vi "Get alarms from PGserver.vi"(6 "conninfo":T1={"host"="localhost", "port"="5432", "client_encoding"="WIN1251", "dbname"="data", "user"="postgres", "password"=""}, 8 "error in":errorcluster, 9 "LevelTable":string[](array[string]), 10 "ALRParamTable":string="f_alr_3", 11 "fcodealr_full":string[](array[string])) -> (0 "error out":errorcluster, 1 "ALRParameters table":u32[][](array[numeric])=[[0, 0, 0, 0, 0, 0, 0], [1, 11, 5000, 5000, 0, 0, 3], [2, 11, 5000, 5000, 0, 2, 3], [3, 11, 5000, 5000, 0, 3, 3], [4, 11, 1000, 0, 0, 4, 0], [5, 1, 5000, 5000, 0, 1, 3], [6, 1, 5000, 5000, 0, 0, 3], [7, 1, 5000, 5000, 0, 2, 3], [8, 1, 5000, 30000, 0, 3, 3], [9, 1, 1000, 0, 0, 4, 0], [10, 2, 5000, 5000, 0, 1, 3], [11, 2, 5000, 5000, 0, 0, 3], [12, 2, 5000, 5000, 0, 2, 3], [13, 2, 5000, 30000, 0, 3, 3], [14, 2, 1000, 0, 0, 4, 0], [15, 10, 5000, 5000, 0, 0, 3], [16, 10, 5000, 5000, 0, 2, 3], [17, 10, 5000, 5000, 0, 3, 3], [18, 10, 1000, 0, 0, 4, 0], [19, 3, 5000, 5000, 0, 2, 3], [20, 3, 5000, 5000, 0, 3, 3], [21, 3, 1000, 0, 0, 4, 0], [22, 4, 5000, 5000, 0, 2, 3], [23, 4, 5000, 5000, 0, 3, 3], [24, 4, 1000, 0, 0, 4, 0], [25, 5, 5000, 5000, 0, 2, 3], [26, 5, 5000, 5000, 0, 3, 3], [27, 5, 1000, 0, 0, 4, 0], [28, 6, 5000, 5000, 0, 2, 3], [29, 6, 1000, 0, 0, 4, 0], [30, 7, 1000, 0, 0, 4, 0], [31, 8, 1000, 0, 0, 4, 0], [32, 9, 5000, 5000, 0, 0, 3]], 2 "ALR type":T3[](array[typedef]), 3 "ALR code":T4[](array[typedef]), 4 "ALRNames":string[][](array[string])=[["", "Перелив в емкости охлажденной воды", "Уровень в емкости охлажденной воды низкий", "Уровень в емкости охлажденной воды аварийно низкий", "Датчик уровня в емкости охлажденной воды неисправен", "Давление после насосов градирни аварийно высокое", "Давление после насосов градирни высокое", "Давление после насосов градирни низкое", "Давление после насосов градирни аварийно низкое", "Датчик давления после насосов градирни неисправен", "Давление перед градирней аварийно высокое", "Давление перед градирней высокое", "Давление перед градирней низкое", "Давление перед градирней аварийно низкое", "Датчик давления перед градирней неисправен", "Перелив в емкости дистиллята", "Уровень в емкости дистиллята низкий", "Уровень в емкости дистиллята аварийно низкий", "Датчик уровеня в емкости дистиллята неисправен", "Давление после насосов дистиллята низкое", "Давление после насосов дистиллята аварийно низкое", "Датчик давления после насосов дистиллята неисправен", "Давление дистиллята перед реактором низкое", "Давление дистиллята перед реактором аварийно низкое", "Датчик давления перед реактором неисправен", "Давление после насоса агломератора низкое", "Давление после насоса агломератора аварийно низкое", "Датчик давления после насоса агломератора неисправен", "Температура после градирни низкая", "Датчик температуры после градирни неисправен", "Датчик температуры перед градирней неисправен", "Датчик температуры дистиллята после насосов неисправен", "Температура дистиллята перед реактором высокая"]], 5 "ALRLevel table":i32[][](array[numeric])=[[0, 0, 0, 0, 0, 0, 0], [1, 11, 5000, 5000, 0, 0, 3], [2, 11, 5000, 5000, 0, 2, 3], [3, 11, 5000, 5000, 0, 3, 3], [4, 11, 1000, 0, 0, 4, 0], [5, 1, 5000, 5000, 0, 1, 3], [6, 1, 5000, 5000, 0, 0, 3], [7, 1, 5000, 5000, 0, 2, 3], [8, 1, 5000, 30000, 0, 3, 3], [9, 1, 1000, 0, 0, 4, 0], [10, 2, 5000, 5000, 0, 1, 3], [11, 2, 5000, 5000, 0, 0, 3], [12, 2, 5000, 5000, 0, 2, 3], [13, 2, 5000, 30000, 0, 3, 3], [14, 2, 1000, 0, 0, 4, 0], [15, 10, 5000, 5000, 0, 0, 3], [16, 10, 5000, 5000, 0, 2, 3], [17, 10, 5000, 5000, 0, 3, 3], [18, 10, 1000, 0, 0, 4, 0], [19, 3, 5000, 5000, 0, 2, 3], [20, 3, 5000, 5000, 0, 3, 3], [21, 3, 1000, 0, 0, 4, 0], [22, 4, 5000, 5000, 0, 2, 3], [23, 4, 5000, 5000, 0, 3, 3], [24, 4, 1000, 0, 0, 4, 0], [25, 5, 5000, 5000, 0, 2, 3], [26, 5, 5000, 5000, 0, 3, 3], [27, 5, 1000, 0, 0, 4, 0], [28, 6, 5000, 5000, 0, 2, 3], [29, 6, 1000, 0, 0, 4, 0], [30, 7, 1000, 0, 0, 4, 0], [31, 8, 1000, 0, 0, 4, 0], [32, 9, 5000, 5000, 0, 0, 3]])   [LabVIEW 2019, in "Alarms.lvlib"]
uses:
  Alarms.lvlib
  Ctl/ALR code.ctl
  Ctl/ALR type.ctl
  Database/ctl/Coninfo.ctl
  Ctl/ALRColumns.ctl
  Database/PostgreSQL2LabVIEW/libpqlv/src/PQfinish.vi
  Database/PostgreSQL2LabVIEW/libpqlv/src/PQconnectdb.vi
  Database/PostgreSQL2LabVIEW/libpqlv/src/PQerrorMessage.vi
  Database/PostgreSQL2LabVIEW/libpqlv/src/PQstatus.vi
  <vilib>/dlg_ctls.llb/Space Constant.vi
  Database/Progress.vi
  Database/PostgreSQL.lvlib
  Database/PostgreSQL2LabVIEW/libpqUtility/libpqutility.lvlib
  Database/PostgreSQL2LabVIEW/libpqUtility64/libpqutility64.lvlib
panel:
  out "PQStatus":T2(ring)
  # "fnum"
  # "alr_ton"
  # "alr_toff"
  # "n_repeat"
  # "fcodealr_full"
  # "alr_name"
  # "fcode_full"
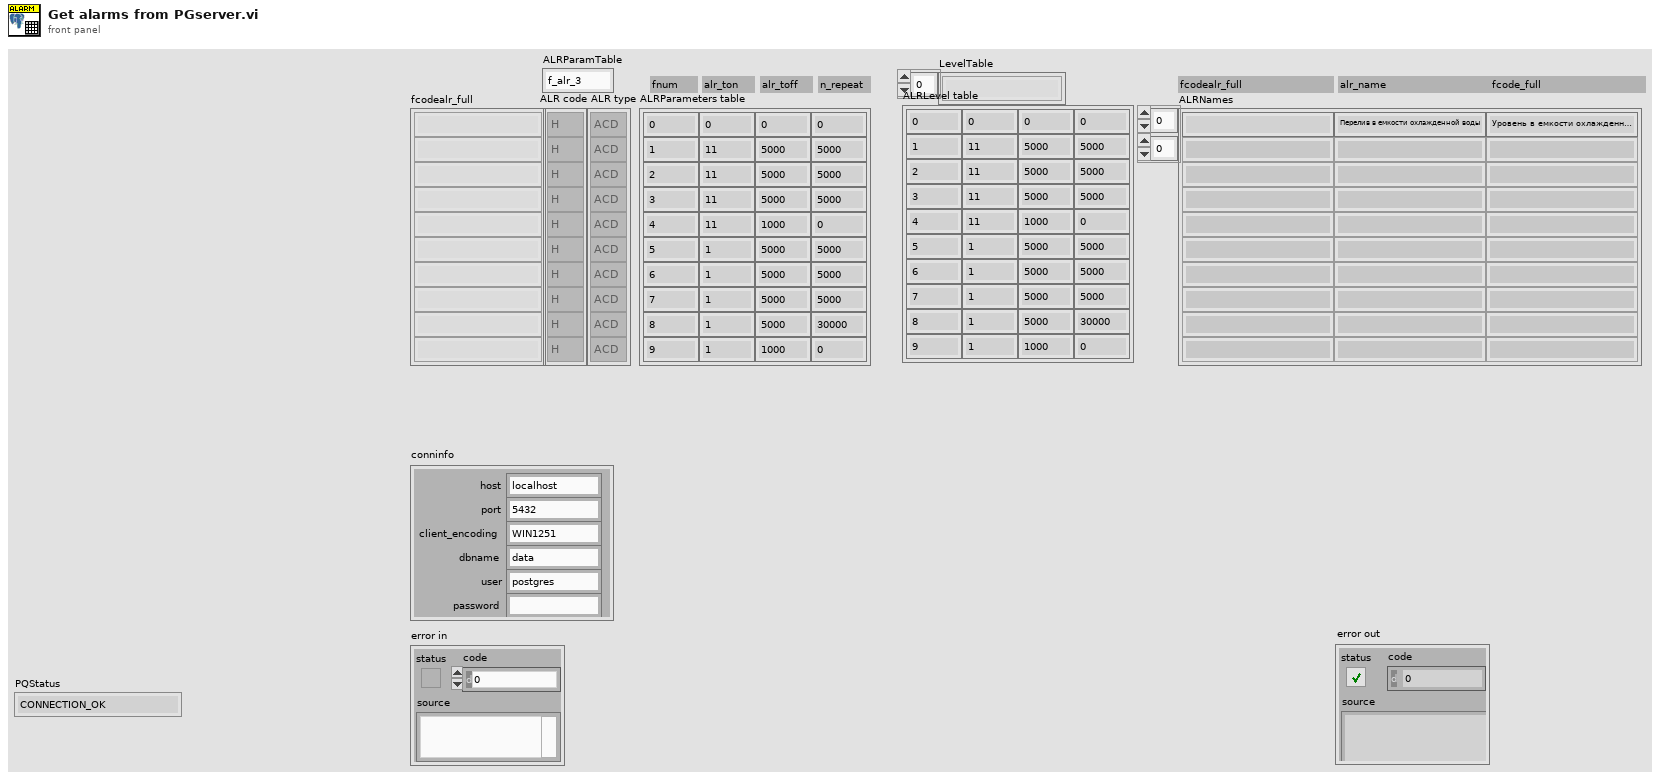
[diagram p1: front panel]
types:
  T1 = typedef "PostgreSQL.lvlib/Coninfo.ctl" = cluster{"host":string, "port":string, "client_encoding":string, "dbname":string, "user":string, "password":string}
  T2 = enum32{"CONNECTION_OK", "CONNECTION_BAD", "CONNECTION_STARTED", "CONNECTION_MADE", "CONNECTION_AWAITING_RESPONSE", "CONNECTION_AUTH_OK", "CONNECTION_SETENV", "CONNECTION_SSL_STARTUP", "CONNECTION_NEEDED"}
  T3 = typedef "Alarms.lvlib/ALR type.ctl" = enum16{"ACD", "ACDR", "ALRN", "ALR"}
  T4 = typedef "Alarms.lvlib/ALR code.ctl" = enum16{"CONN", "H", "HH", "L", "LL", "SERR", "ON", "OFF", "XM19", "XM24", "XM47", "XM51", "XM52", "XM53", "XM54", "XM55", "XM56", "XM61", "XM62", "XM63", "XM64", "XM65", "XM66"}
  T5 = typedef "Alarms.lvlib/ALRColumns.ctl" = enum16{"alr_ton", "alr_toff", "n_repeat", "fcodealr", "alr_type", "alrname", "fcode_full"}
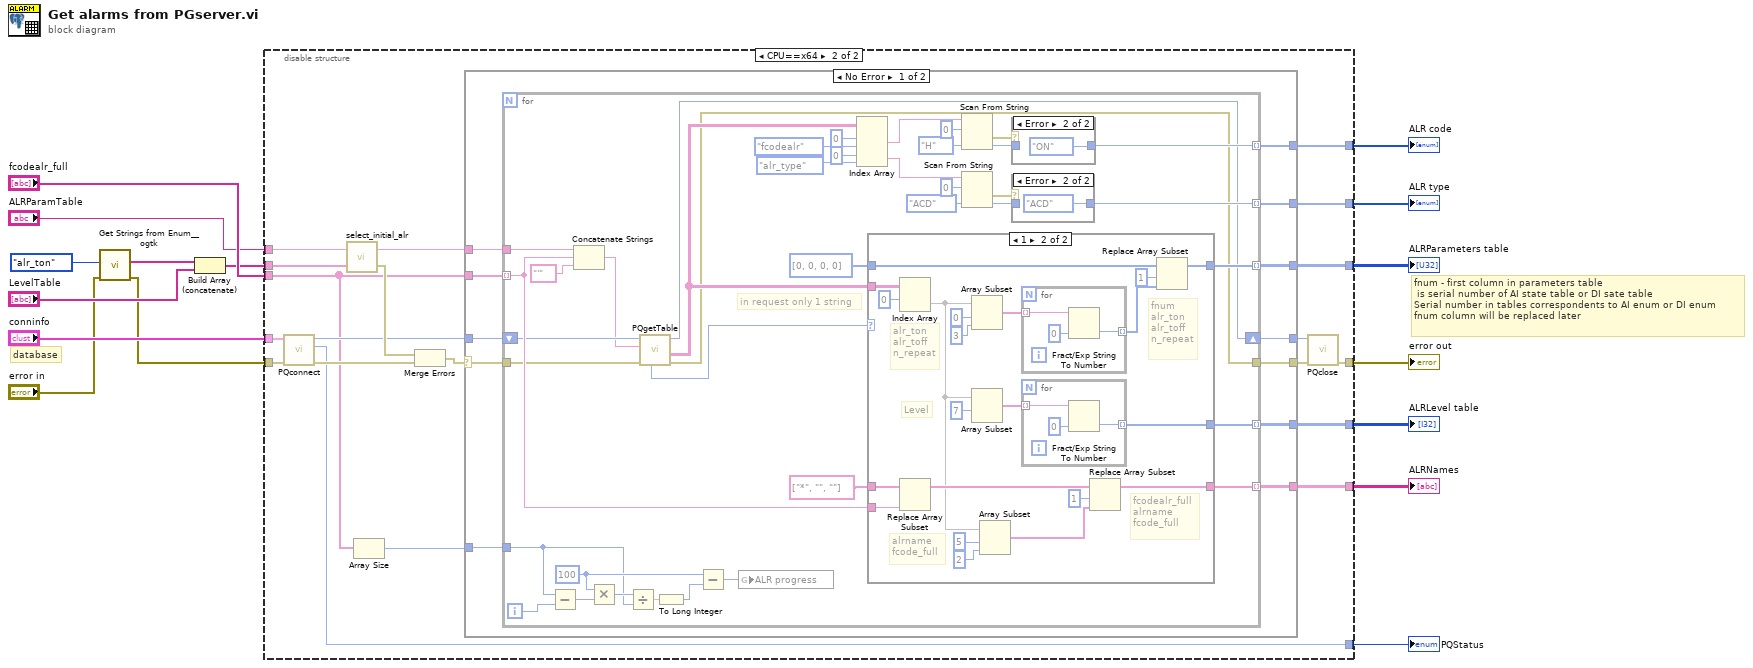
[diagram p0: block diagram]
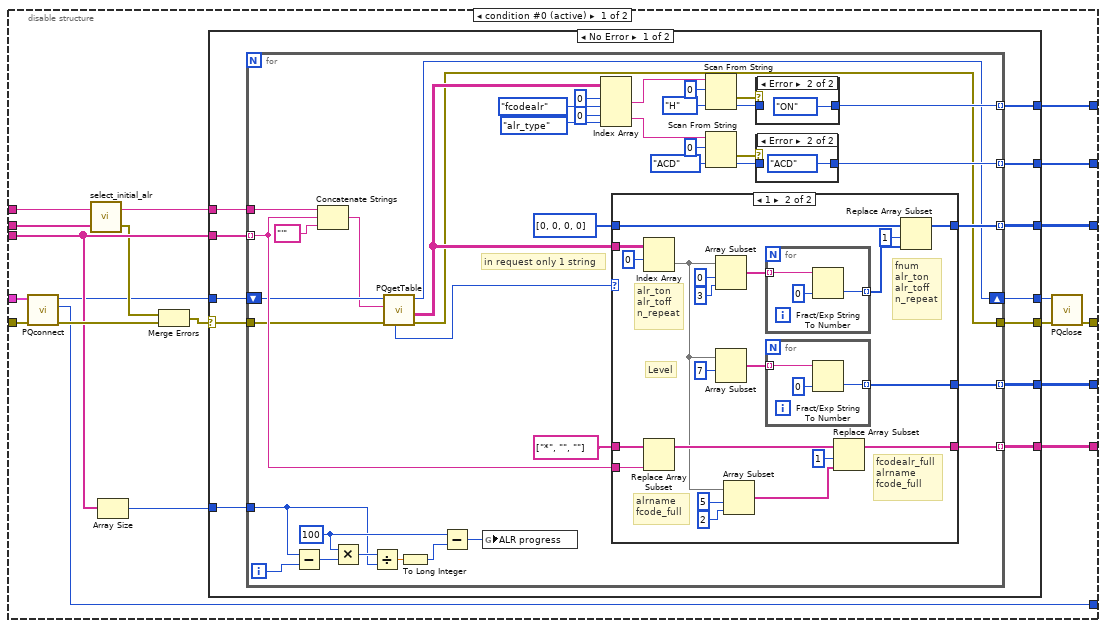
[diagram p2: hidden frame]
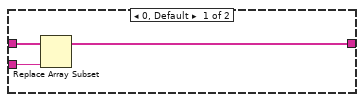
[diagram p3: hidden frame]
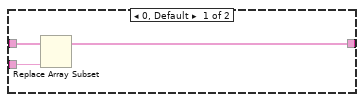
[diagram p7: hidden frame]
diagram:
  # "fnum - first column in parameters table\n is serial number of AI state table or DI sate table\nSerial number in tables correspondents to AI enum or DI enum\nfnum column will be replaced later"
  # "database"
  n1 = call <userlib>:"Get Strings from Enum__ogtk.vi"("error in (no error)"="error in", "Enum"=ALRColumns."alr_ton" ("ALRColumns")) -> ("error out"=w2:errorcluster, "Enum Strings"=w1:string[])  [unwired: 6 in, 2 out]
  n2 = Build Array (concatenate)(w1, "LevelTable") -> (w7:string[])
  n3 = disable-structure shown="CPU==x64" {
    disable-tunnel: "fcodealr_full" -> [w35 w133]
    disable-tunnel: [w34 w126] -> w15
    disable-tunnel: "ALRParamTable" -> [w33 w135]
    disable-tunnel: [w32 w125] -> w13
    disable-tunnel: [w31 w124] -> w12
    disable-tunnel: [w30 w127] -> w11
    disable-tunnel: [w29 w129] -> w10
    disable-tunnel: "conninfo" -> [w28 w132]
    disable-tunnel: w2 -> [w26 w131]
    disable-tunnel: w7 -> [w25 w134]
    disable-tunnel: [w24 w128] -> w6
    disable-tunnel: [w23 w130] -> w5
    frame condition #0 (active) {
      n4 = call "PQconnect.vi"("error in (no error)"=w26, "conninfo"=w28) -> ("error out"=w36:errorcluster, "PQStatus"=w23:T2, "conn"=w18:u32)  [unwired: 7 in]
      n5 = call "select_initial_alr.vi"("Column table"=w25, "table"=w33) -> ("Data to write"=w20:errorcluster, "parameters"=w21:string)
      n6 = Array Size(array=w35) -> (size(s)=w22:i32)
      n7 = Merge Errors(w20, w36) -> (w19:errorcluster)
      n8 = case shown="No Error" w19 {
        selector: w19 -> [w46 w123]
        tunnel: w35 -> [w44 _]
        tunnel: [w48 _] -> w34
        tunnel: [w47 _] -> w29
        tunnel: w22 -> [w45 _]
        tunnel: w18 -> [w43 w122]
        tunnel: w21 -> [w42 _]
        tunnel: [w41 _] -> w31
        tunnel: [w40 _] -> w32
        tunnel: [w39 w123] -> w27
        tunnel: [w38 _] -> w24
        tunnel: [w37 w122] -> w17
        frame No Error {
          n9 = for {
            tunnel: [w65] -> w47 mode=indexing
            tunnel: [w62] -> w48 mode=indexing
            tunnel: w46 -> [w56]
            tunnel: w45 -> [w78]
            tunnel: w44 -> [w61] mode=indexing
            tunnel: w42 -> [w87]
            tunnel: [w64] -> w41 mode=indexing
            tunnel: [w63] -> w40 mode=indexing
            tunnel: [w54] -> w39
            tunnel: [w52] -> w38 mode=indexing
            shift-right: [w51] -> w37
            shift-left: w43 -> [w58]
            i -> [w79]
            w83 = 100 ("y")
            # "in request only 1 string"
            n10 = Subtract(x=w78, y=w79) -> (x-y=w82:i32)
            n11 = Concatenate Strings(w87, w61, "'" ("table")) -> (w57:string)
            n12 = Multiply(x=w83, y=w82) -> (x*y=w85:i32)
            n13 = Divide(x=w85, y=w78) -> (x/y=w81:dbl)
            n14 = call "PQgetTable.vi"("error in"=w56, "query"=w57, "conn"=w58) -> ("error out"=w54:errorcluster, "Data"=w55:string[][], "conn_out"=w51:u32, "PQnTuples"=w53:i32)  [unwired: 4 in, 1 out]
            n15 = To Long Integer(number=w81) -> (32bit integer=w80:i32)
            n16 = Subtract(x=w83, y=w80) -> (x-y=w84:i32)
            n17 = global write "Progress.vi" "ALR progress"(w84) -> ()
            n18 = Index Array(array=w55, index (row) #1=0 ("disabled index (row)"), index (col) #1=ALRColumns."fcodealr" ("ALRColumns"), index (row) #2=0 ("disabled index (row)"), index (col) #2=ALRColumns."alr_type" ("ALRColumns")) -> (element #1=w74:string, element #2=w68:string)
            n19 = case shown="1" w53 {
              tunnel: [_ w98] -> w62
              tunnel: w55 -> [_ w111]
              tunnel: [w88 w102] -> w65
              tunnel: w61 -> [w90 w106]
              tunnel: string[] ["*", "", ""] ("appended array") -> [w89 w107]
              tunnel: u32[] [0, 0, 0, 0] ("appended array") -> [_ w101]
              tunnel: [_ w91] -> w52
              frame 0, Default {
                n20 = Replace Array Subset(array=w89, new element=w90) -> (w88:string[])  [unwired: 1 in]
              }
              frame 1 {
                # "fnum\nalr_ton\nalr_toff\nn_repeat"
                # "fcodealr_full\nalrname\nfcode_full"
                # "alrname\nfcode_full"
                # "Level"
                # "alr_ton\nalr_toff\nn_repeat"
                n21 = Index Array(array=w111, index (row)=0) -> (element=w93:string[])  [unwired: 1 in]
                n22 = Replace Array Subset(array=w107, new element=w106) -> (w105:string[])  [unwired: 1 in]
                n23 = Array Subset(array=w93, index=0, length=3) -> (w95:string[])
                n24 = Array Subset(array=w93, index=7) -> (w92:string[])  [unwired: 1 in]
                n25 = Array Subset(array=w93, index=5, length=2) -> (w104:string[])
                n26 = for {
                  tunnel: w95 -> [w117] mode=indexing
                  tunnel: [w116] -> w99 mode=indexing
                  n27 = Fract/Exp String To Number(string=w117, default (0 dbl)=u32 0 ("String")) -> (number=w116:u32)  [unwired: 2 in, 1 out]
                }
                n28 = for {
                  tunnel: w92 -> [w114] mode=indexing
                  tunnel: [w113] -> w91 mode=indexing
                  n29 = Fract/Exp String To Number(string=w114, default (0 dbl)=0 ("String")) -> (number=w113:i32)  [unwired: 2 in, 1 out]
                }
                n30 = Replace Array Subset(array=w105, new element=w104, index=1) -> (w102:string[])
                n31 = Replace Array Subset(array=w101, new element=w99, index=1) -> (w98:u32[])
              }
            }
            n32 = Scan From String(input string=w74, initial scan location=u32 0, default 1=ALR_code."H" ("ALR code")) -> (error out=w77:errorcluster, output 1=w73:T4)  [unwired: 2 in, 2 out]
            n33 = Scan From String(input string=w68, initial scan location=u32 0, default 1=ALR_type."ACD" ("ALR type")) -> (error out=w70:errorcluster, output 1=w72:T3)  [unwired: 2 in, 2 out]
            n34 = case shown="Error" w77 {
              tunnel: w73 -> [w120 _]
              tunnel: [w120 ALR_code."ON" ("ALR code")] -> w64
              frame No Error {
              }
              frame Error {
              }
            }
            n35 = case shown="Error" w70 {
              tunnel: w72 -> [w118 _]
              tunnel: [w118 ALR_type."ACD" ("ALR type")] -> w63
              frame No Error {
              }
              frame Error {
              }
            }
          }
        }
        frame Error {
        }
      }
      n36 = call "PQclose.vi"("error in (no error)"=w27, "conn"=w17) -> ("error out"=w30:errorcluster)  [unwired: 9 in]
    }
    frame condition #1 {
      n37 = call "PQconnect.vi"("error in (no error)"=w131, "conninfo"=w132) -> ("error out"=w143:errorcluster, "PQStatus"=w130:T2, "conn"=w137:u64)  [unwired: 7 in]
      n38 = call "select_initial_alr.vi"("Column table"=w134, "table"=w135) -> ("Data to write"=w139:errorcluster, "parameters"=w140:string)
      n39 = Array Size(array=w133) -> (size(s)=w141:i32)
      n40 = Merge Errors(w139, w143) -> (w138:errorcluster)
      n41 = case shown="No Error" w138 {
        selector: w138 -> [w153 w230]
        tunnel: w133 -> [w151 _]
        tunnel: [w155 _] -> w126
        tunnel: [w154 _] -> w129
        tunnel: w141 -> [w152 _]
        tunnel: w137 -> [w150 w229]
        tunnel: w140 -> [w149 _]
        tunnel: [w148 _] -> w124
        tunnel: [w147 _] -> w125
        tunnel: [w146 w230] -> w142
        tunnel: [w145 _] -> w128
        tunnel: [w144 w229] -> w136
        frame No Error {
          n42 = for {
            tunnel: [w172] -> w154 mode=indexing
            tunnel: [w169] -> w155 mode=indexing
            tunnel: w153 -> [w163]
            tunnel: w152 -> [w185]
            tunnel: w151 -> [w168] mode=indexing
            tunnel: w149 -> [w194]
            tunnel: [w171] -> w148 mode=indexing
            tunnel: [w170] -> w147 mode=indexing
            tunnel: [w161] -> w146
            tunnel: [w159] -> w145 mode=indexing
            shift-right: [w158] -> w144
            shift-left: w150 -> [w165]
            i -> [w186]
            w190 = 100 ("y")
            # "in request only 1 string"
            n43 = Subtract(x=w185, y=w186) -> (x-y=w189:i32)
            n44 = Concatenate Strings(w194, w168, "'" ("table")) -> (w164:string)
            n45 = Multiply(x=w190, y=w189) -> (x*y=w192:i32)
            n46 = Divide(x=w192, y=w185) -> (x/y=w188:dbl)
            n47 = call "PQgetTable.vi"("error in"=w163, "query"=w164, "conn"=w165) -> ("error out"=w161:errorcluster, "Data"=w162:string[][], "conn_out"=w158:u64, "PQnTuples"=w160:i64)  [unwired: 4 in, 1 out]
            n48 = To Long Integer(number=w188) -> (32bit integer=w187:i32)
            n49 = Subtract(x=w190, y=w187) -> (x-y=w191:i32)
            n50 = global write "Progress.vi" "ALR progress"(w191) -> ()
            n51 = Index Array(array=w162, index (row) #1=0 ("disabled index (row)"), index (col) #1=ALRColumns."fcodealr" ("ALRColumns"), index (row) #2=0 ("disabled index (row)"), index (col) #2=ALRColumns."alr_type" ("ALRColumns")) -> (element #1=w181:string, element #2=w175:string)
            n52 = case shown="1" w160 {
              tunnel: [_ w205] -> w169
              tunnel: w162 -> [_ w218]
              tunnel: [w195 w209] -> w172
              tunnel: w168 -> [w197 w213]
              tunnel: string[] ["*", "", ""] ("appended array") -> [w196 w214]
              tunnel: u32[] [0, 0, 0, 0] ("appended array") -> [_ w208]
              tunnel: [_ w198] -> w159
              frame 0, Default {
                n53 = Replace Array Subset(array=w196, new element=w197) -> (w195:string[])  [unwired: 1 in]
              }
              frame 1 {
                # "fnum\nalr_ton\nalr_toff\nn_repeat"
                # "fcodealr_full\nalrname\nfcode_full"
                # "alrname\nfcode_full"
                # "Level"
                # "alr_ton\nalr_toff\nn_repeat"
                n54 = Index Array(array=w218, index (row)=0) -> (element=w200:string[])  [unwired: 1 in]
                n55 = Replace Array Subset(array=w214, new element=w213) -> (w212:string[])  [unwired: 1 in]
                n56 = Array Subset(array=w200, index=0, length=3) -> (w202:string[])
                n57 = Array Subset(array=w200, index=7) -> (w199:string[])  [unwired: 1 in]
                n58 = Array Subset(array=w200, index=5, length=2) -> (w211:string[])
                n59 = for {
                  tunnel: w202 -> [w224] mode=indexing
                  tunnel: [w223] -> w206 mode=indexing
                  n60 = Fract/Exp String To Number(string=w224, default (0 dbl)=u32 0 ("String")) -> (number=w223:u32)  [unwired: 2 in, 1 out]
                }
                n61 = for {
                  tunnel: w199 -> [w221] mode=indexing
                  tunnel: [w220] -> w198 mode=indexing
                  n62 = Fract/Exp String To Number(string=w221, default (0 dbl)=0 ("String")) -> (number=w220:i32)  [unwired: 2 in, 1 out]
                }
                n63 = Replace Array Subset(array=w212, new element=w211, index=1) -> (w209:string[])
                n64 = Replace Array Subset(array=w208, new element=w206, index=1) -> (w205:u32[])
              }
            }
            n65 = Scan From String(input string=w181, initial scan location=u32 0, default 1=ALR_code."H" ("ALR code")) -> (error out=w184:errorcluster, output 1=w180:T4)  [unwired: 2 in, 2 out]
            n66 = Scan From String(input string=w175, initial scan location=u32 0, default 1=ALR_type."ACD" ("ALR type")) -> (error out=w177:errorcluster, output 1=w179:T3)  [unwired: 2 in, 2 out]
            n67 = case shown="Error" w184 {
              tunnel: w180 -> [w227 _]
              tunnel: [w227 ALR_code."ON" ("ALR code")] -> w171
              frame No Error {
              }
              frame Error {
              }
            }
            n68 = case shown="Error" w177 {
              tunnel: w179 -> [w225 _]
              tunnel: [w225 ALR_type."ACD" ("ALR type")] -> w170
              frame No Error {
              }
              frame Error {
              }
            }
          }
        }
        frame Error {
        }
      }
      n69 = call "PQclose.vi"("error in (no error)"=w142, "conn"=w136) -> ("error out"=w127:errorcluster)  [unwired: 9 in]
    }
  }
  "error out" <- w11
  "ALRParameters table" <- w15
  "ALRNames" <- w10
  "ALR code" <- w12
  "ALR type" <- w13
  "ALRLevel table" <- w6
  "PQStatus" <- w5
